vi "NI 9215_task.vi"(1 "Samples per channel":i32=1000, 2 "sample mode":i32(ring)=10178 items=["Finite Samples"=10178, "Continuous Samples"=10123, "Hardware Timed Single Point"=12522], 3 "MODULE 5 (0-10V)":string="CDR_AI", 4 "Sample Rate":dbl=1000.0 format="%0.2f", 5 "error in":errorcluster) -> (14 "task out":refnum<k21>, 19 "error out":errorcluster)   [LabVIEW 2019]
uses:
  <vilib>/DAQmx/configure/timing.llb/DAQmx Timing (Sample Clock).vi
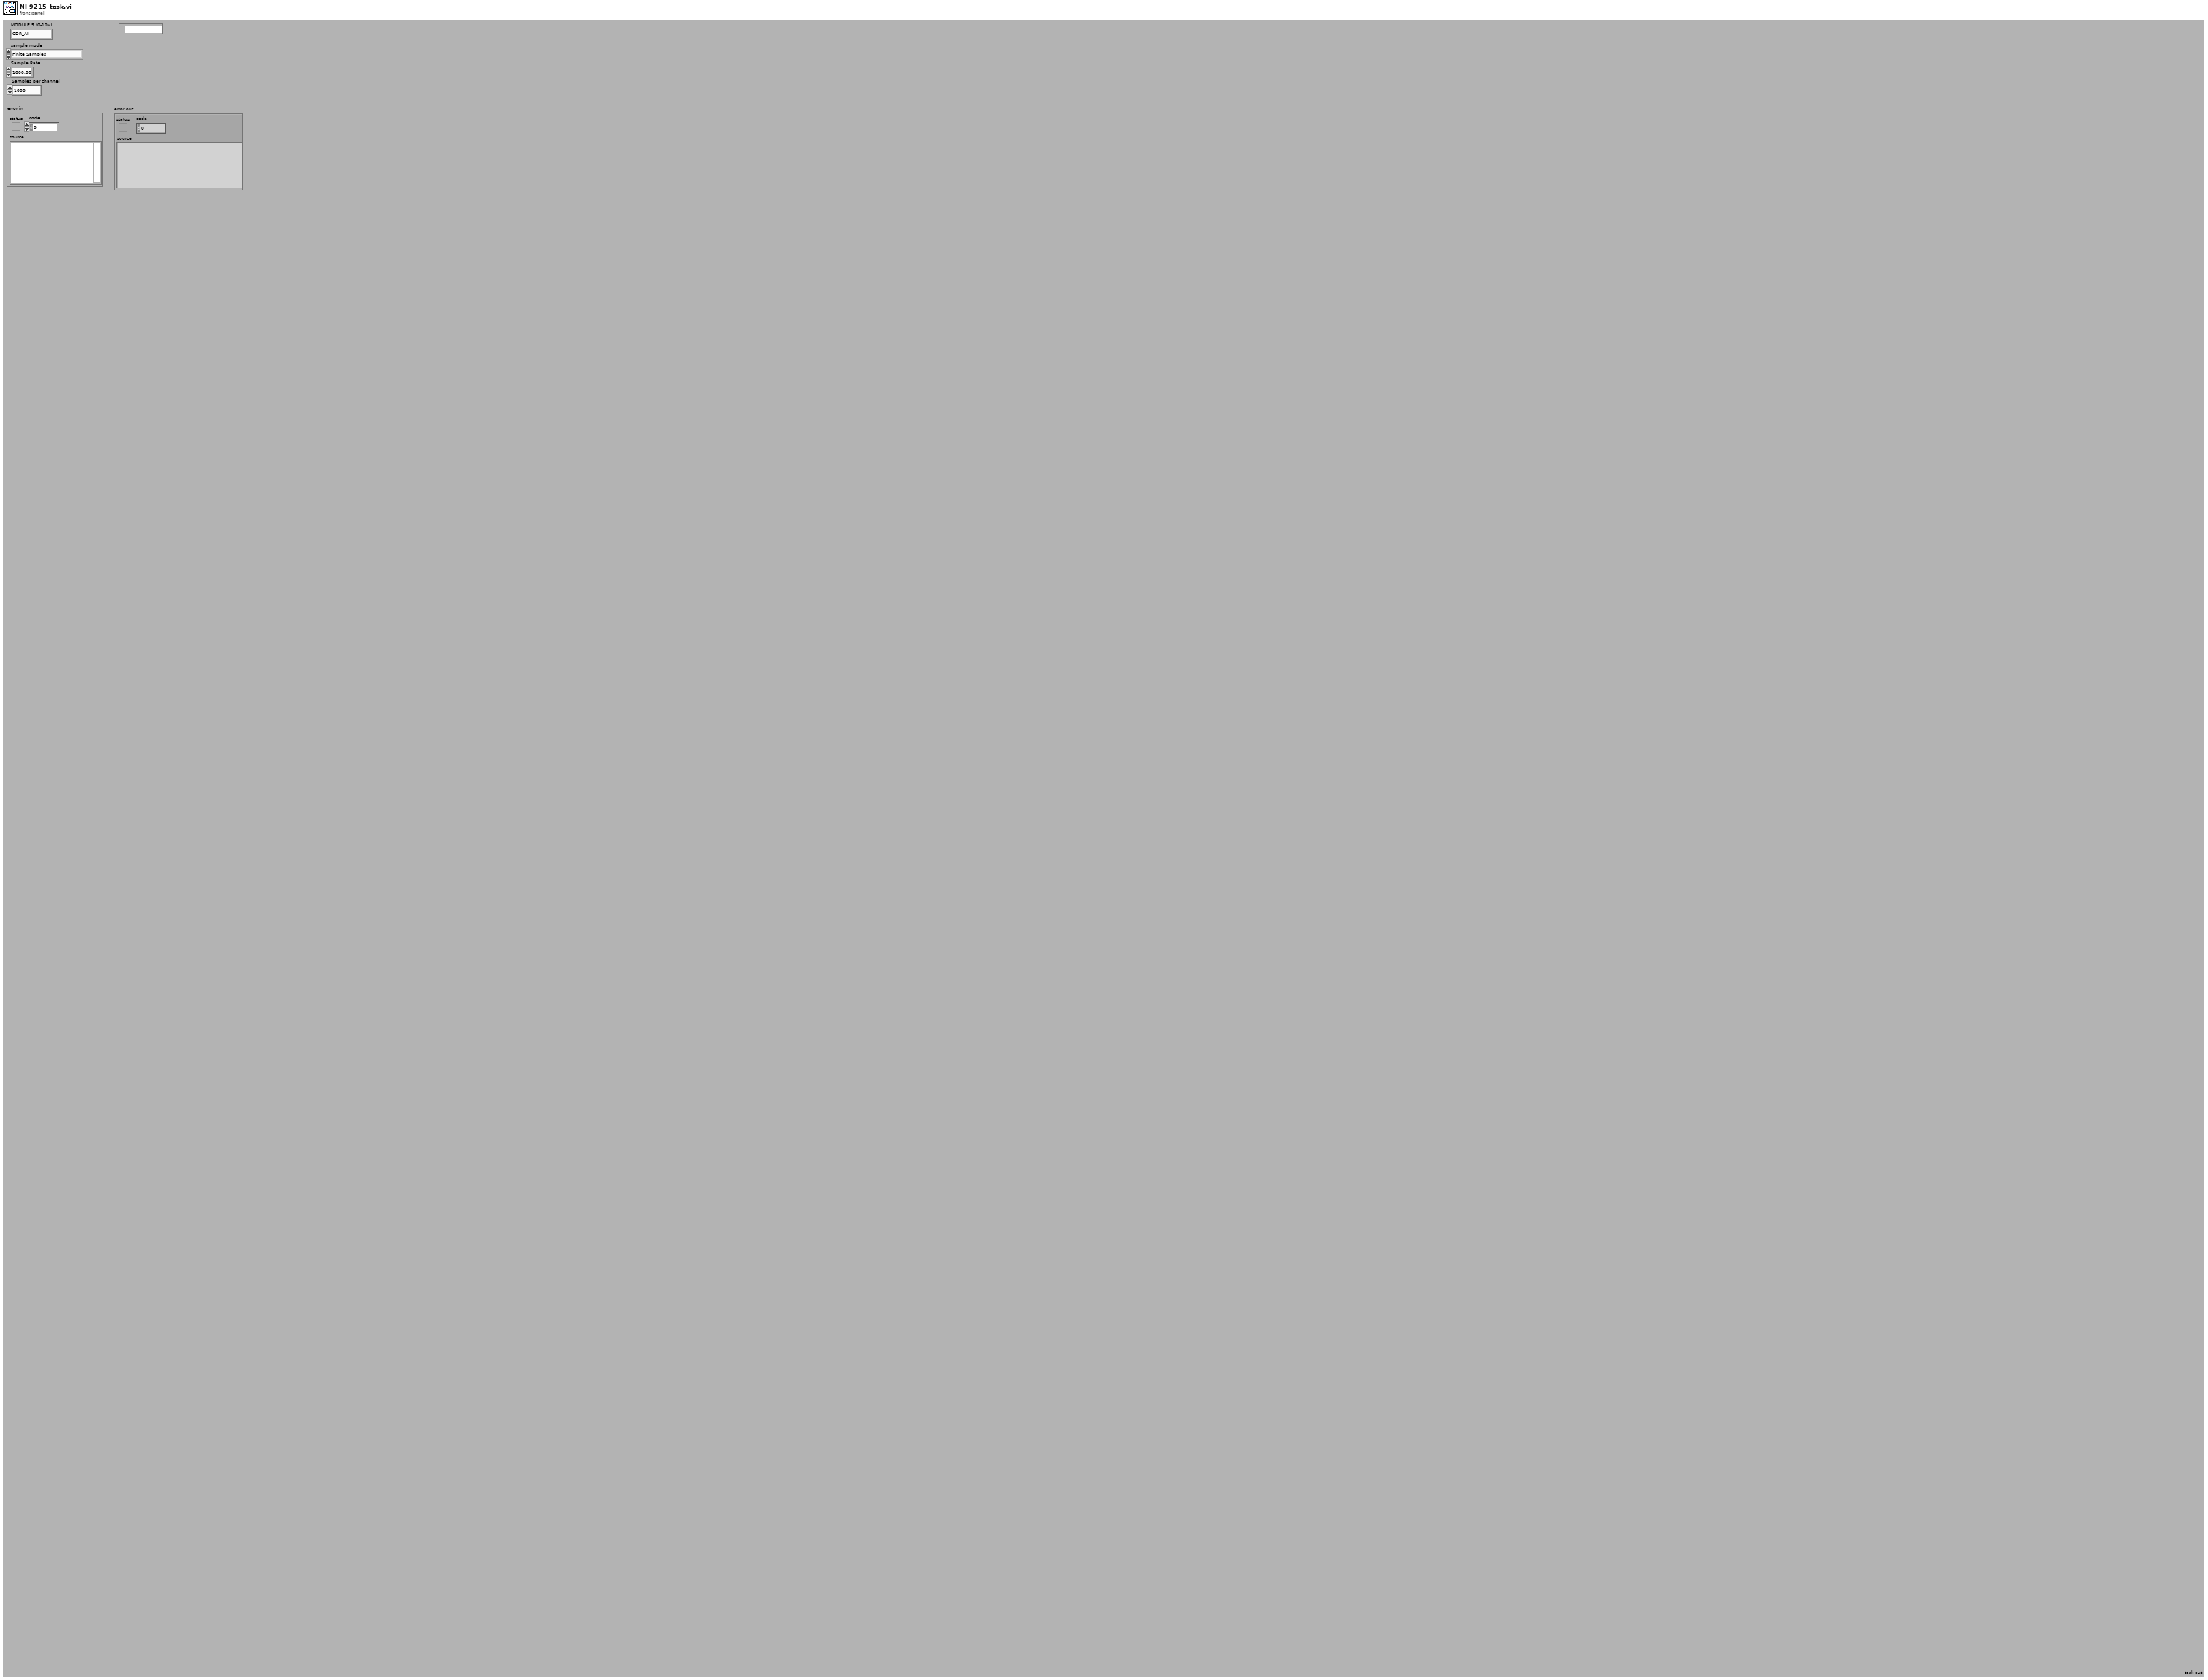
[diagram p1: front panel]
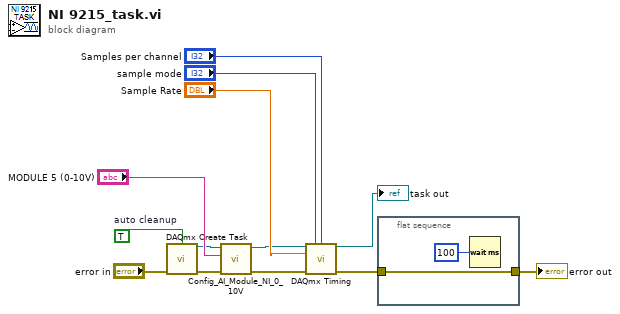
[diagram p0: block diagram]
diagram:
  w12 = TRUE  # auto cleanup
  n1 = call <vilib>:"DAQmx Create Task.vi"("auto cleanup"=w12, "error in"="error in") -> ("task out"=w3:refnum<k21>, "error out"=w2:errorcluster)  [unwired: 12 in]
  n2 = call "Config_AI_Module_NI_0_10V.vi"("error in (no error)"=w2, "MODULE NAME"="MODULE 5 (0-10V)", "Refnum in"=w3) -> ("error out"=w5:errorcluster, "Refnum out"=w4:refnum<k21>)  [unwired: 7 in]
  n3 = call-poly <vilib>:"DAQmx Timing.vi"("task/channels in"=w4, "sample mode"="sample mode", "samples per channel"="Samples per channel", "rate"="Sample Rate", "error in"=w5) -> ("task out"=→"task out":refnum<k21>, "error out"=w8:errorcluster)  [unwired: 9 in]
  n4 = flat-sequence {
    tunnel: [w14] -> w7
    tunnel: w8 -> [w14]
    frame #0 {
      n5 = Wait (ms)(milliseconds to wait=u32 100) -> ()  [unwired: 1 out]
    }
  }
  "error out" <- w7
